vi "LoadFileOptions.vi"(8 "error in (no error)":errorcluster, 9 "Item Ref in":T1 format="%.0x", 10 "Directory In":refnum<vi>, 11 "Filename in":refnum<vi>) -> (0 "error out":errorcluster, 3 "Item Ref out":T1 format="%.0x")   [LabVIEW 2024, in "Embedded TDMS Logger System Explorer.lvlib"]
doc: "Load the file options - i.e. filename and directory from the System Definition for the Main Page UI."
uses:
  Embedded TDMS Logger System Explorer.lvlib
  <vilib>/NI VeriStand/Custom Device API/Custom Device Item Ref.ctl
  <vilib>/NI VeriStand/Custom Device API/Get Item Property (String).vi
  <vilib>/NI VeriStand/Custom Device API/Set Item Property (String).vi
  <vilib>/NI VeriStand/Custom Device API/Custom Device API.lvlib
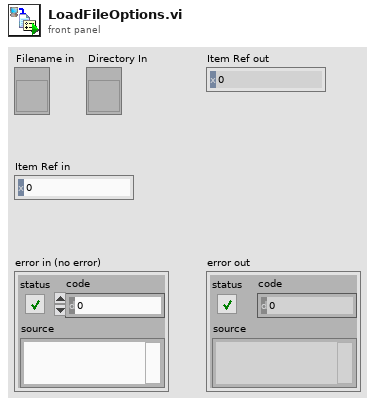
[diagram p1: front panel]
types:
  T1 = typedef "Custom Device API.lvlib/Custom Device Item Ref.ctl" = u64
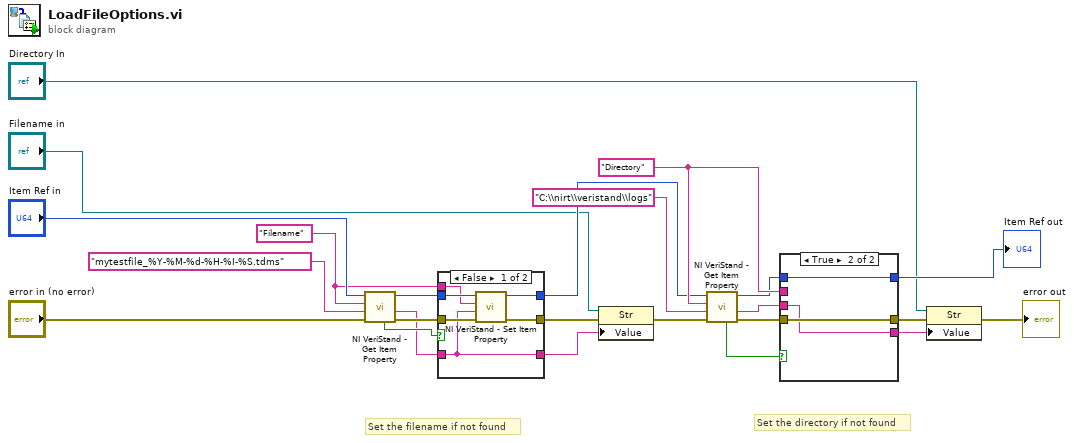
[diagram p0: block diagram]
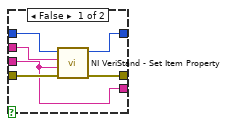
[diagram p3: hidden frame]
diagram:
  w1 = "Filename"
  w23 = "Directory"
  # "Set the directory if not found"
  # "Set the filename if not found"
  n1 = call-poly <vilib>:"NI VeriStand - Get Item Property.vi"("error in (no error)"="error in (no error)", "Default Value"="mytestfile_%Y-%M-%d-%H-%I-%S.tdms", "Property Name"=w1, "Item Ref in"="Item Ref in") -> ("error out"=w10:errorcluster, "Value"=w8:string, "Item Ref out"=w9:T1, "Found?"=w11:bool)  [unwired: 4 in]
  n2 = case shown="False" w11 {
    tunnel: [w30 w33] -> w4
    tunnel: w9 -> [w29 w33]
    tunnel: [w28 w32] -> w12
    tunnel: w10 -> [w27 w32]
    tunnel: w8 -> [w26 w31]
    tunnel: [w26 w31] -> w13
    tunnel: w1 -> [w25 _]
    frame False {
      n3 = call-poly <vilib>:"NI VeriStand - Set Item Property.vi"("error in (no error)"=w27, "Value"=w26, "Property Name"=w25, "Item Ref in"=w29) -> ("error out"=w28:errorcluster, "Item Ref out"=w30:T1)  [unwired: 5 in, 1 out]
    }
    frame True {
    }
  }
  n4 = property class="Str"(reference="Filename in", error in=w12, "Value"=w13) -> (error out=w3:errorcluster)  [unwired: 1 out]
  n5 = call-poly <vilib>:"NI VeriStand - Get Item Property.vi"("error in (no error)"=w3, "Default Value"="C:\\nirt\\veristand\\logs", "Property Name"=w23, "Item Ref in"=w4) -> ("error out"=w19:errorcluster, "Value"=w21:string, "Item Ref out"=w20:T1, "Found?"=w18:bool)  [unwired: 4 in]
  n6 = case shown="True" w18 {
    tunnel: [w39 w42] -> w24
    tunnel: w20 -> [w38 w42]
    tunnel: [w37 w41] -> w17
    tunnel: w19 -> [w36 w41]
    tunnel: w21 -> [w34 w40]
    tunnel: [w34 w40] -> w16
    tunnel: w23 -> [w35 _]
    frame False {
      n7 = call-poly <vilib>:"NI VeriStand - Set Item Property.vi"("error in (no error)"=w36, "Value"=w34, "Property Name"=w35, "Item Ref in"=w38) -> ("error out"=w37:errorcluster, "Item Ref out"=w39:T1)  [unwired: 5 in, 1 out]
    }
    frame True {
    }
  }
  "Item Ref out" <- w24
  n8 = property class="Str"(reference="Directory In", error in=w17, "Value"=w16) -> (error out=→"error out":errorcluster)  [unwired: 1 out]
